vi "Robot Drive Teleop.vi"(0 "Controller Mode":enum16{"X-Box Controller", "Joysticks"}(ring), 1 "Drive Mode":enum16{"Tank Drive", "Arcade Drive"}(ring), 2 "RobotDriveDevRef":T3={"DevStatus"={"status"=FALSE, "code"=0, "source"=""}, "Motors[]"=[], "Square Inputs"=FALSE, "Max Output"=1.0}, 3 "Joystick0DevRef":T1={"Device"=enum."USB 1"}, 4 "Joystick1DevRef":T1={"Device"=enum."USB 1"}) -> (5 "Motor Values":dbl[](array[numeric]))   [LabVIEW 2015]
uses:
  <vilib>/Rock Robotics/WPI/RobotDrive/WPI_RobotDriveDevRef.ctl
  <vilib>/Rock Robotics/WPI/MotorControl/WPI_MotorControlDeviceRef.ctl
  <vilib>/Rock Robotics/WPI/MotorControl/WPI_MotorControlType.ctl
  <vilib>/Rock Robotics/SystemInterfaces/DIO/FPGA_DIOPWMChannel.ctl
  <vilib>/Rock Robotics/WPI/PWM/WPI_PWMDeadband.ctl
  <vilib>/Rock Robotics/WPI/CAN/Jaguar/SubVIs/WPI_CANJaguar_ControlMode.ctl
  <vilib>/Rock Robotics/WPI/CAN/TalonSRX/WPI_CANTalonSRX_APIControlMode.ctl
  <vilib>/Rock Robotics/WPI/Joystick/WPI_JoystickDevRef.ctl
  <vilib>/Rock Robotics/WPI/Joystick/WPI_JoystickDeviceEnum.ctl
panel:
  in  "Axes (Joystick 1)":dbl[](array[numeric])
  in  "Axes (Joystick 0)":dbl[](array[numeric])
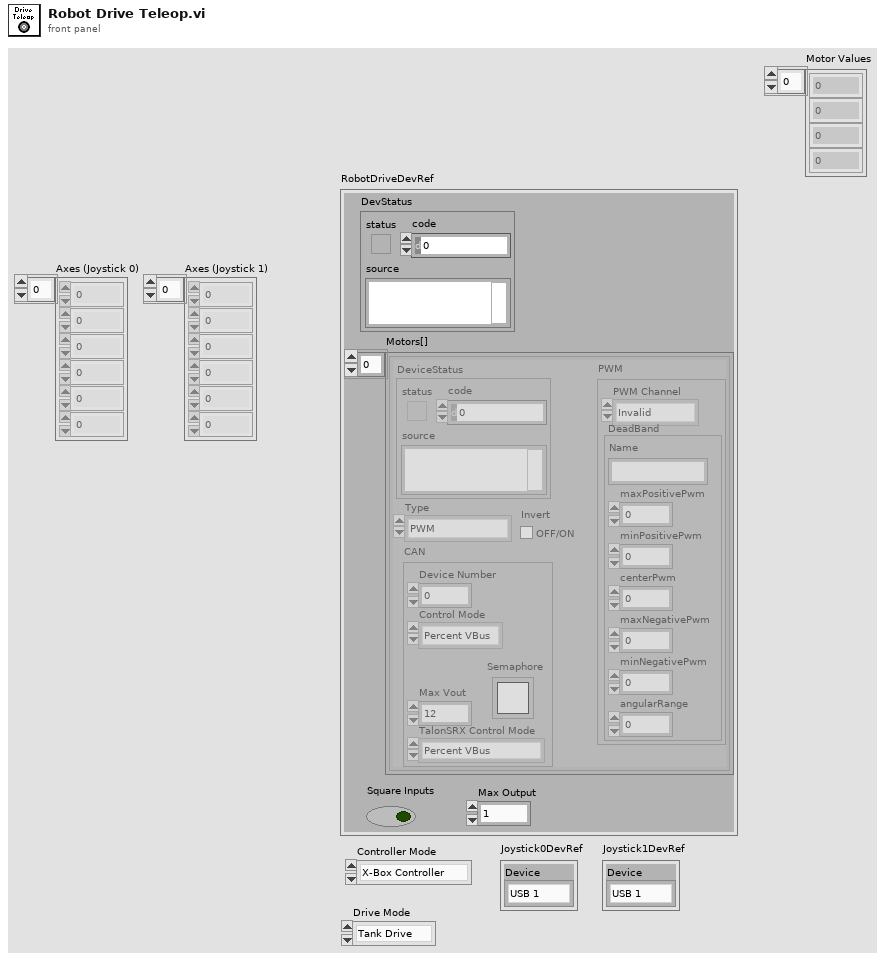
[diagram p1: front panel]
types:
  T1 = typedef "WPI_JoystickDevRef.ctl" = cluster{"Device":T2}
  T2 = typedef "WPI_JoystickDeviceEnum.ctl" = enum16{"USB 0", "USB 1", "USB 2", "USB 3", "USB 4", "USB 5"}
  T3 = typedef "WPI_RobotDriveDevRef.ctl" = cluster{"DevStatus":errorcluster, "Motors[]":T4[], "Square Inputs":bool, "Max Output":dbl}
  T4 = typedef "WPI_MotorControlDeviceRef.ctl" = cluster{"DeviceStatus":errorcluster, "Type":T5, "PWM":cluster{"PWM Channel":T6, "DeadBand":T7}, "CAN":cluster{"Device Number":u8, "Control Mode":T8, "Semaphore":T9, "Max Vout":dbl, "TalonSRX Control Mode":T10}, "Invert":bool}
  T5 = typedef "WPI_MotorControlType.ctl" = enum16{"PWM", "CAN", "CANTalonSRX"}
  T6 = typedef "FPGA_DIOPWMChannel.ctl" = enum8{"PWM 0", "PWM 1", "PWM 2", "PWM 3", "PWM 4", "PWM 5", "PWM 6", "PWM 7", "PWM 8", "PWM 9", "PWM MXP 0", "PWM MXP 1", "PWM MXP 2", "PWM MXP 3", "PWM MXP 4", "PWM MXP 5", "PWM MXP 6", "PWM MXP 7", "PWM MXP 8", "PWM MXP 9", "Invalid"}
  T7 = typedef "WPI_PWMDeadband.ctl" = cluster{"Name":string, "maxPositivePwm":i32, "minPositivePwm":i32, "centerPwm":i32, "maxNegativePwm":i32, "minNegativePwm":i32, "angularRange":u16}
  T8 = typedef "WPI_CANJaguar_ControlMode.ctl" = enum8{"Percent VBus", "Current", "Speed", "Position", "Voltage"}
  T9 = typedef "Semaphore RefNum" = refnum<k1>
  T10 = typedef "WPI_CANTalonSRX_APIControlMode.ctl" = enum8{"Percent VBus", "Speed", "Position", "Slave", "Unchanged / Invalid", "Voltage Compensation", "Current", "Motion Profile"}
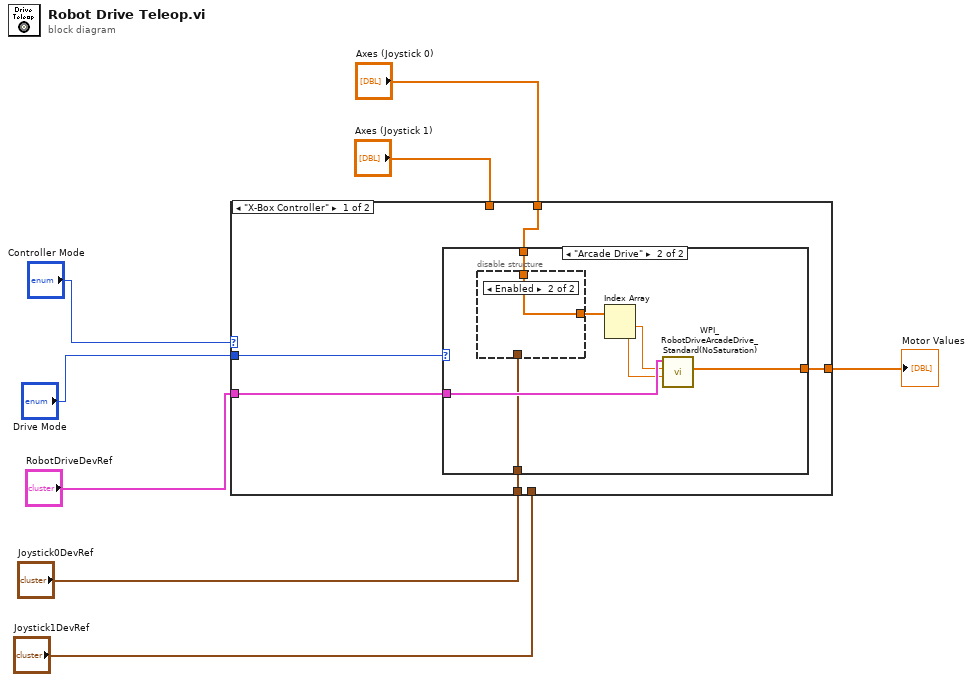
[diagram p0: block diagram]
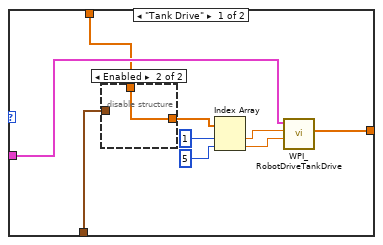
[diagram p2: hidden frame]
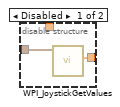
[diagram p3: hidden frame]
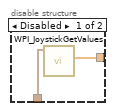
[diagram p4: hidden frame]
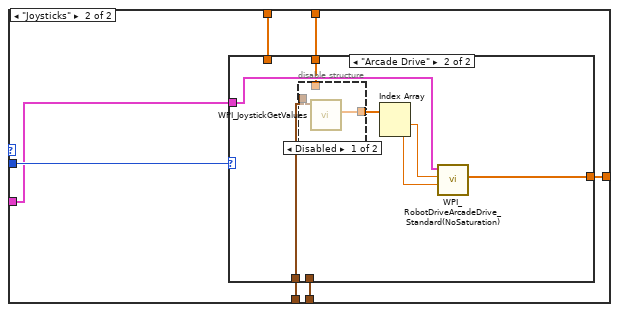
[diagram p5: hidden frame]
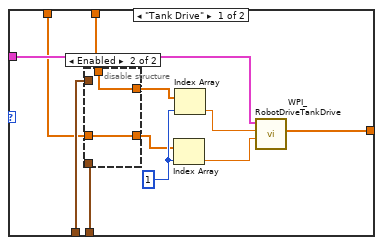
[diagram p6: hidden frame]
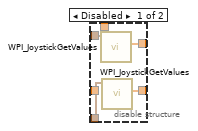
[diagram p7: hidden frame]
diagram:
  n1 = case shown="\"X-Box Controller\"" "Controller Mode" {
    tunnel: "Drive Mode" -> [w13 w42]
    tunnel: "RobotDriveDevRef" -> [w12 w39]
    tunnel: "Joystick0DevRef" -> [w11 w41]
    tunnel: [w10 w38] -> w4
    tunnel: "Joystick1DevRef" -> [_ w40]
    tunnel: "Axes (Joystick 0)" -> [w9 w37]
    tunnel: "Axes (Joystick 1)" -> [_ w36]
    frame "X-Box Controller" {
      n2 = case shown="\"Arcade Drive\"" w13 {
        tunnel: w12 -> [w18 w32]
        tunnel: w11 -> [w22 w30]
        tunnel: [w15 w27] -> w10
        tunnel: w9 -> [w14 w26]
        frame "Tank Drive" {
          n3 = disable-structure shown="Enabled" {
            disable-tunnel: w22 -> [w24 _]
            disable-tunnel: [w23 w25] -> w19
            disable-tunnel: w14 -> [_ w25]
            frame Disabled {
              n4 = call <vilib>:"WPI_JoystickGetValues.vi"("JoystickDevRef"=w24) -> ("Axes"=w23:dbl[])  [unwired: 6 in, 4 out]
            }
            frame Enabled {
            }
          }
          n5 = Index Array(array=w19, index #1=1 ("index"), index #2=5 ("index")) -> (element #1=w17:dbl, element #2=w16:dbl)
          n6 = call <vilib>:"WPI_RobotDriveTankDrive.vi"("Right axis value"=w16, "Left axis value"=w17, "RobotDriveDevRef"=w18) -> ("Motor Values"=w15:dbl[])  [unwired: 6 in, 2 out]
        }
        frame "Arcade Drive" {
          n7 = disable-structure shown="Enabled" {
            disable-tunnel: [w34 w35] -> w31
            disable-tunnel: w30 -> [w33 _]
            disable-tunnel: w26 -> [_ w35]
            frame Disabled {
              n8 = call <vilib>:"WPI_JoystickGetValues.vi"("JoystickDevRef"=w33) -> ("Axes"=w34:dbl[])  [unwired: 6 in, 4 out]
            }
            frame Enabled {
            }
          }
          n9 = Index Array(array=w31) -> (element #1=w29:dbl, element #2=w28:dbl)  [unwired: 2 in]
          n10 = call <vilib>:"WPI_RobotDriveArcadeDrive_Standard(NoSaturation).vi"("Y axis value"=w28, "X axis value"=w29, "RobotDriveDevRef"=w32) -> ("Motor Values"=w27:dbl[])  [unwired: 1 in, 7 out]
        }
      }
    }
    frame "Joysticks" {
      n11 = case shown="\"Arcade Drive\"" w42 {
        tunnel: w41 -> [w53 w62]
        tunnel: w40 -> [w52 _]
        tunnel: w39 -> [w48 w63]
        tunnel: [w45 w61] -> w38
        tunnel: w37 -> [w44 w60]
        tunnel: w36 -> [w43 _]
        frame "Tank Drive" {
          w51 = 1
          n12 = disable-structure shown="Enabled" {
            disable-tunnel: w53 -> [w57 _]
            disable-tunnel: w52 -> [w56 _]
            disable-tunnel: [w55 w59] -> w50
            disable-tunnel: [w54 w58] -> w49
            disable-tunnel: w44 -> [_ w59]
            disable-tunnel: w43 -> [_ w58]
            frame Disabled {
              n13 = call <vilib>:"WPI_JoystickGetValues.vi"("JoystickDevRef"=w57) -> ("Axes"=w55:dbl[])  [unwired: 6 in, 4 out]
              n14 = call <vilib>:"WPI_JoystickGetValues.vi"("JoystickDevRef"=w56) -> ("Axes"=w54:dbl[])  [unwired: 6 in, 4 out]
            }
            frame Enabled {
            }
          }
          n15 = Index Array(array=w49, index=w51) -> (element=w46:dbl)
          n16 = Index Array(array=w50, index=w51) -> (element=w47:dbl)
          n17 = call <vilib>:"WPI_RobotDriveTankDrive.vi"("Right axis value"=w46, "Left axis value"=w47, "RobotDriveDevRef"=w48) -> ("Motor Values"=w45:dbl[])  [unwired: 6 in, 2 out]
        }
        frame "Arcade Drive" {
          n18 = disable-structure shown="Disabled" {
            disable-tunnel: [w68 w69] -> w66
            disable-tunnel: w62 -> [w67 _]
            disable-tunnel: w60 -> [_ w69]
            frame Disabled {
              n19 = call <vilib>:"WPI_JoystickGetValues.vi"("JoystickDevRef"=w67) -> ("Axes"=w68:dbl[])  [unwired: 6 in, 4 out]
            }
            frame Enabled {
            }
          }
          n20 = Index Array(array=w66) -> (element #1=w65:dbl, element #2=w64:dbl)  [unwired: 2 in]
          n21 = call <vilib>:"WPI_RobotDriveArcadeDrive_Standard(NoSaturation).vi"("Y axis value"=w64, "X axis value"=w65, "RobotDriveDevRef"=w63) -> ("Motor Values"=w61:dbl[])  [unwired: 1 in, 7 out]
        }
      }
    }
  }
  "Motor Values" <- w4
